vi "IMAQ-Device2Cluster.vi"(1 "errorImage IN":errorcluster, 2 "Image IN":T1) -> (0 "Image Device OUT":cluster{"Image":T1, "errorImage":errorcluster})   [LabVIEW 2010]
uses:
  <vilib>/vision/Image Controls.llb/IMAQ Image.ctl
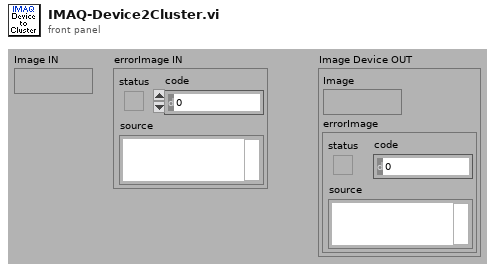
[diagram p1: front panel]
types:
  T1 = typedef "IMAQ Image.ctl" = refnum<image>
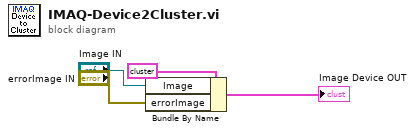
[diagram p0: block diagram]
diagram:
  n1 = Bundle By Name(cluster=cluster{"Image":T1, "errorImage":errorcluster} {"Image"=refnum, "errorImage"={"status"=FALSE, "code"=0, "source"=""}} ("Image Device IN"), "Image"="Image IN", "errorImage"="errorImage IN") -> (→"Image Device OUT":cluster{"Image":T1, "errorImage":errorcluster})
